vi "_Set 1 DAC Value.vi"(1 "DAC":u32, 3 "Ch#":u8) -> (0 "PIC Monitor":u8)   [LabVIEW 2015]
uses:
  Type/_FPGA Chip Type.ctl
  <vilib>/rvi/eio/common/nirviEmuTemplateMethod_errors.vi
  <vilib>/rvi/Memory/Memory_Emulation/nirvimemoryEmulation.vi
  <vilib>/rvi/Memory/Memory_Emulation/nirvimemoryFastEmulation.vi
  <vilib>/rvi/DataTransferAndStorage/Container/Common/niFpgaContainerGetUniqueNameForEmu.vi
  <vilib>/rvi/Memory/Memory_Emulation/niFpgaMemoryEmulationCacheClearOnFirstRun.vi
  <vilib>/rvi/Memory/Memory_Emulation/nirvimemoryEmulationManagerCache_MakeExclusive.vi
  <vilib>/rvi/Memory/Memory_Emulation/niFpgaMemoryEmulationValidateCache.vi
  <vilib>/rvi/Memory/Memory_Emulation/nirvimemoryEmulationManagerCache_InsertValue.vi
  <vilib>/Utility/error.llb/Clear Errors.vi
  <vilib>/rvi/Memory/Memory_Emulation/nirvimemoryEmulationManagerCache_ReleaseExclusive.vi
  <vilib>/rvi/Memory/Memory_Emulation/nirvimemoryEmulationManagerCache_GetValue.vi
  <vilib>/rvi/Emulation/niFpgaEmulationIsFPGAContextNoSignature.vi
  <vilib>/rvi/Emulation/niFpgaSctlEmulationGetInTimedLoop.vi
  <vilib>/rvi/Memory/Memory_Emulation/nirvimemoryEmulationManagerCache_SetValue.vi
  <vilib>/rvi/Emulation/niFpgaSctlEmulationResourceMgr.vi
  <vilib>/eio/EIONode/EIONode.xnode
  <vilib>/rvi/DataTransferAndStorage/Container/XNode/niFpgaContainer.xnode
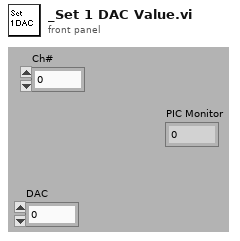
[diagram p1: front panel]
types:
  T1 = typedef "_FPGA Chip Type.ctl" = enum8{"None", "ADC1", "ADC2", "ADC3", "ADC4", "ADC5", "ADC6", "ADC7", "ADC8", "ADC9", "ADC10", "ADC11", "ADC12", "ADC13", "DAC1", "DAC2", "DAC3", "DAC4", "DAC5", "LENS1", "LENS2", "LENS3", "LENS4", "LENS5", "LENS6", "LENS7", "MASS1", "MASS2", "MASS3", "MASS4", "MASS5", "OSC1", "OSC2", "OSC3", "LATCH1", "LATCH2", "LATCH3", "LATCH4", "PIC1", "PIC2", "PIC3", "PIC4"}
  T2 = cluster{"Boolean array[0]":bool, "Boolean array[1]":bool, "Boolean array[2]":bool, "Boolean array[3]":bool, "Boolean array[4]":bool, "Boolean array[5]":bool, "Boolean array[6]":bool, "Boolean array[7]":bool, "Boolean array[8]":bool, "Boolean array[9]":bool, "Boolean array[10]":bool, "Boolean array[11]":bool, "Boolean array[12]":bool, "Boolean array[13]":bool, "Boolean array[14]":bool, "Boolean array[15]":bool, "Boolean array[16]":bool, "Boolean array[17]":bool, "Boolean array[18]":bool, "Boolean array[19]":bool, "Boolean array[20]":bool, "Boolean array[21]":bool, "Boolean array[22]":bool, "Boolean array[23]":bool, "Boolean array[24]":bool, "Boolean array[25]":bool, "Boolean array[26]":bool, "Boolean array[27]":bool, "Boolean array[28]":bool, "Boolean array[29]":bool, "Boolean array[30]":bool, "Boolean array[31]":bool}
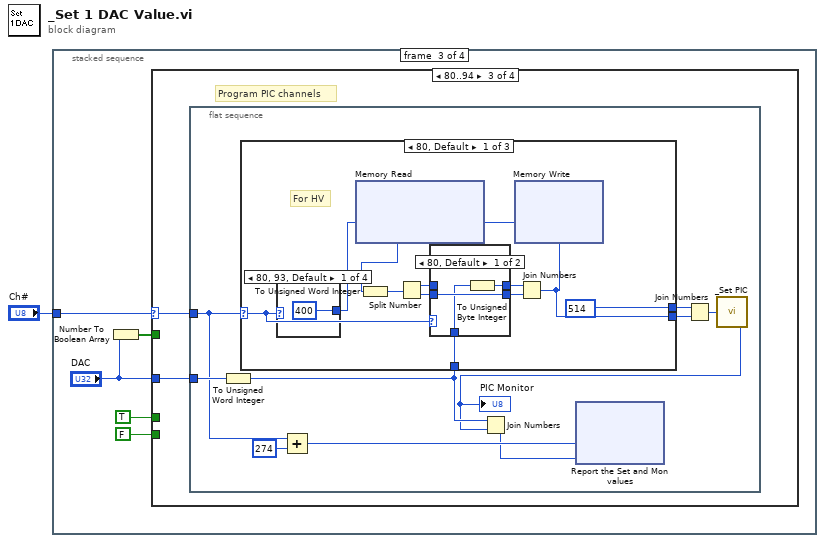
[diagram p0: block diagram]
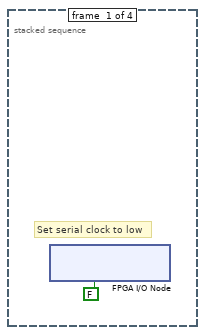
[diagram p2: hidden frame]
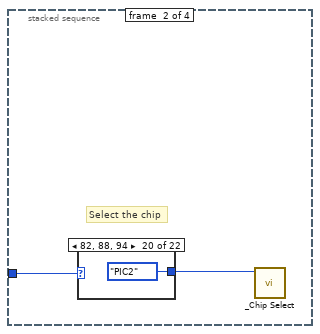
[diagram p3: hidden frame]
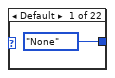
[diagram p4: hidden frame]
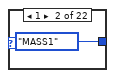
[diagram p5: hidden frame]
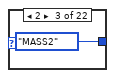
[diagram p6: hidden frame]
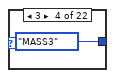
[diagram p7: hidden frame]
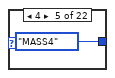
[diagram p8: hidden frame]
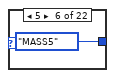
[diagram p9: hidden frame]
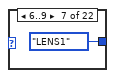
[diagram p10: hidden frame]
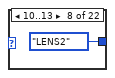
[diagram p11: hidden frame]
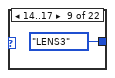
[diagram p12: hidden frame]
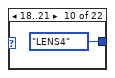
[diagram p13: hidden frame]
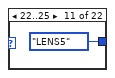
[diagram p14: hidden frame]
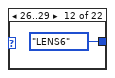
[diagram p15: hidden frame]
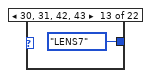
[diagram p16: hidden frame]
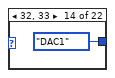
[diagram p17: hidden frame]
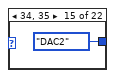
[diagram p18: hidden frame]
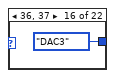
[diagram p19: hidden frame]
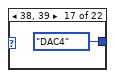
[diagram p20: hidden frame]
diagram:
  n1 = stacked-sequence {
    tunnel: "Ch#" -> [_ w3 w30 _]
    frame #0 {
      # "Set serial clock to low"
      n2 = xnode "FPGA I/O Node"("Digtal IO/DIO9"=FALSE ("Port1/DIO0")) -> ()  [unwired: 1 in, 1 out]
    }
    frame #1 {
      # "Select the chip"
      n3 = case shown="82, 88, 94" w3 {
        tunnel: [_FPGA_Chip_Type."None" ("ChipType") _FPGA_Chip_Type."MASS1" ("ChipType") _FPGA_Chip_Type."MASS2" ("ChipType") _FPGA_Chip_Type."MASS3" ("ChipType") _FPGA_Chip_Type."MASS4" ("ChipType") _FPGA_Chip_Type."MASS5" ("ChipType") _FPGA_Chip_Type."LENS1" ("ChipType") _FPGA_Chip_Type."LENS2" ("ChipType") _FPGA_Chip_Type."LENS3" ("ChipType") _FPGA_Chip_Type."LENS4" ("ChipType") _FPGA_Chip_Type."LENS5" ("ChipType") _FPGA_Chip_Type."LENS6" ("ChipType") _FPGA_Chip_Type."LENS7" ("ChipType") _FPGA_Chip_Type."DAC1" ("ChipType") _FPGA_Chip_Type."DAC2" ("ChipType") _FPGA_Chip_Type."DAC3" ("ChipType") _FPGA_Chip_Type."DAC4" ("ChipType") _FPGA_Chip_Type."DAC5" ("ChipType") _FPGA_Chip_Type."PIC1" ("ChipType") _FPGA_Chip_Type."PIC2" ("ChipType") _FPGA_Chip_Type."PIC3" ("ChipType") _FPGA_Chip_Type."PIC4" ("ChipType")] -> w4
        frame Default {
        }
        frame 1 {
        }
        frame 2 {
        }
        frame 3 {
        }
        frame 4 {
        }
        frame 5 {
        }
        frame 6..9 {
        }
        frame 10..13 {
        }
        frame 14..17 {
        }
        frame 18..21 {
        }
        frame 22..25 {
        }
        frame 26..29 {
        }
        frame 30, 31, 42, 43 {
        }
        frame 32, 33 {
        }
        frame 34, 35 {
        }
        frame 36, 37 {
        }
        frame 38, 39 {
        }
        frame 40, 41 {
        }
        frame 80, 81, 87, 93 {
        }
        frame 82, 88, 94 {
        }
        frame 83, 84, 89, 91 {
        }
        frame 85, 86, 90, 92 {
        }
      }
      n4 = call "_Chip Select.vi"("ChipType"=w4) -> ()  [unwired: 1 in, 6 out]
    }
    frame #2 {
      n5 = Number To Boolean Array(number="DAC") -> (Boolean array=w29:bool[])
      n6 = case shown="80..94" w30 {
        selector: w30 -> [w32 w69 w96 _]
        tunnel: w29 -> [w35 w74 _ _]
        tunnel: TRUE -> [w34 w72 _ _]
        tunnel: FALSE -> [w33 w71 _ _]
        tunnel: "DAC" -> [_ _ w95 _]
        frame 1..31, 42, 43 {
          n7 = flat-sequence {
            tunnel: w35 -> [w36]
            tunnel: w32 -> [w61]
            tunnel: w34 -> [w38]
            tunnel: w33 -> [w37]
            frame #0 {
              # "D17"
              # "D0"
              # "WR"
              # "A1"
              # "A0"
              # "2 Address bits"
              # "Program Parallel DAC Data"
              n8 = case shown="1, Default" w61 {
                tunnel: w38 -> [w62 _ w65 w66]
                tunnel: w37 -> [_ w63 w64 w67]
                tunnel: [w62 w63 w65 w67] -> w40
                tunnel: [w62 w63 w64 w66] -> w39
                frame 1, Default {
                  # "A = 3"
                }
                frame 6, 10, 14, 18, 22, 26, 30 {
                  # "A = 0"
                }
                frame 7, 11, 15, 19, 23, 27, 31 {
                  # "A = 1"
                }
                frame 8, 12, 16, 20, 24, 28, 42 {
                  # "A = 2"
                }
              }
              n9 = call "Wait"("Count(Ticks)"=u8 3) -> ()  [unwired: 1 out]
              n10 = Array To Cluster(array=w36) -> (cluster=w42:T2)
              n11 = Unbundle By Name(w42) -> ("Boolean array[0]"=w43:bool, "Boolean array[1]"=w44:bool, "Boolean array[2]"=w45:bool, "Boolean array[3]"=w46:bool, "Boolean array[4]"=w47:bool, "Boolean array[5]"=w48:bool, "Boolean array[6]"=w49:bool, "Boolean array[7]"=w50:bool, "Boolean array[8]"=w51:bool, "Boolean array[9]"=w52:bool, "Boolean array[10]"=w53:bool, "Boolean array[11]"=w54:bool, "Boolean array[12]"=w55:bool, "Boolean array[13]"=w56:bool, "Boolean array[14]"=w57:bool, "Boolean array[15]"=w58:bool, "Boolean array[16]"=w59:bool, "Boolean array[17]"=w60:bool)
              n12 = xnode "FPGA I/O Node"("Digtal IO/DIO42"=w43, "Digtal IO/DIO41"=w44, "Digtal IO/DIO40"=w45, "Digtal IO/DIO39"=w46, "Digtal IO/DIO38"=w47, "Digtal IO/DIO37"=w48, "Digtal IO/DIO36"=w49, "Digtal IO/DIO35"=w50, "Digtal IO/DIO34"=w51, "Digtal IO/DIO32"=w52, "Digtal IO/DIO31"=w53, "Digtal IO/DIO30"=w54, "Digtal IO/DIO29"=w55, "Digtal IO/DIO28"=w56, "Digtal IO/DIO27"=w57, "Digtal IO/DIO26"=w58, "Digtal IO/DIO25"=w59, "Digtal IO/DIO24"=w60, "Digtal IO/DIO62"=w40, "Digtal IO/DIO61"=w39, "Digtal IO/DIO64"=w37) -> ()  [unwired: 21 in, 21 out]
            }
            frame #1 {
              # "Reset WR bit"
              n13 = xnode "FPGA I/O Node"("Digtal IO/DIO64"=TRUE) -> ()  [unwired: 1 in, 1 out]
            }
          }
        }
        frame 32..41 {
          # "Serial DAC updated immediately without waiting for LDAC"
          # "Transmit the last bit first"
          # "4 Control bits"
          # "Remove the last 16 bits"
          # "R0"
          # "PWR"
          # "SPD"
          # "R1"
          # "Program Serial DAC Data"
          n14 = flat-sequence {
            tunnel: w72 -> [w81]
            tunnel: w71 -> [w80]
            tunnel: w70 -> [w79]
            frame #0 {
              n15 = call "_Update Serial DAC.vi"() -> ()  [unwired: 4 in, 4 out]
            }
            frame #1 {
              n16 = for {
                shift-right: [w83] -> w82
                shift-left: w80 -> [w84]
                tunnel: w79 -> [w83] mode=indexing
                tunnel: w81 -> [w85]
                n17 = flat-sequence {
                  tunnel: w85 -> [w87]
                  tunnel: w84 -> [w86]
                  tunnel: w83 -> [w88]
                  frame #0 {
                    n18 = call "_Update Serial DAC.vi"("DIN (F)"=w86, "Clock (F)"=w87) -> ()  [unwired: 2 in, 4 out]
                  }
                  frame #1 {
                    n19 = call "_Update Serial DAC.vi"("DIN (F)"=w88) -> ()  [unwired: 3 in, 4 out]
                  }
                }
              }
              n20 = call "_Update Serial DAC.vi"("DIN (F)"=w82, "Clock (F)"=w81) -> ()  [unwired: 2 in, 4 out]
            }
          }
          n21 = case shown="32, 34, 36, 38, 40" w69 {
            tunnel: [w91 w94] -> w75
            tunnel: w72 -> [w90 w93]
            tunnel: w71 -> [w89 w92]
            frame 33, Default {
              # "Update DAC B"
              n22 = Build Array(w89, w89, w90, w89) -> (w91:bool[])
            }
            frame 32, 34, 36, 38, 40 {
              # "Update DAC A"
              n23 = Build Array(w92, w92, w93, w93) -> (w94:bool[])
            }
          }
          n24 = Array Subset(array=w74, length=16 ("index")) -> (w76:bool[])  [unwired: 1 in]
          n25 = Replace Array Subset(array=w76, new element=w75, index=12) -> (w73:bool[])
          n26 = Reverse 1D Array(array=w73) -> (reversed array=w70:bool[])
        }
        frame 80..94 {
          # "Program PIC channels"
          n27 = flat-sequence {
            tunnel: w96 -> [w97]
            tunnel: w95 -> [w101]
            frame #0 {
              n28 = To Unsigned Word Integer(number=w101) -> (unsigned 16bit integer=w100:u16)
              n29 = case shown="80, Default" w97 {
                selector: w97 -> [w117 _ _]
                tunnel: [i16 514 i16 257 i16 771] -> w106
                tunnel: [w114 w128 u16 0] -> w104
                tunnel: w100 -> [w115 w128 _]
                frame 80, Default {
                  # "For HV"
                  n30 = case shown="80, 93, Default" w117 {
                    tunnel: [u16 400 u16 401 u16 402 u16 403] -> w111
                    frame 80, 93, Default {
                    }
                    frame 82, 94 {
                    }
                    frame 83, 91 {
                    }
                    frame 85, 92 {
                    }
                  }
                  n31 = xnode ("Memory Read")("Address"=w111) -> ("Data"=w108:u32)  [unwired: 1 in, 1 out]
                  n32 = To Unsigned Word Integer(number=w108) -> (unsigned 16bit integer=w107:u16)
                  n33 = Split Number(x=w107) -> (hi(x)=w113:u8, lo(x)=w112:u8)
                  n34 = case shown="80, Default" w117 {
                    tunnel: w113 -> [_ w123]
                    tunnel: w112 -> [w120 _]
                    tunnel: [w120 w121] -> w109
                    tunnel: [w118 w123] -> w110
                    tunnel: w115 -> [w119 w122]
                    frame 80, Default {
                      n35 = To Unsigned Byte Integer(number=w119) -> (unsigned 8bit integer=w118:u8)
                    }
                    frame 91..94 {
                      n36 = To Unsigned Byte Integer(number=w122) -> (unsigned 8bit integer=w121:u8)
                    }
                  }
                  n37 = Join Numbers(hi=w110, lo=w109) -> ((hi.lo)=w114:u16)
                  n38 = xnode ("Memory Write")("Address"=w111, "Data"=w114) -> ()  [unwired: 1 in, 1 out]
                }
                frame 81, 84, 86 {
                  # "for Temp"
                }
                frame 87..90 {
                  # "for Probe ID"
                }
              }
              n39 = Add(x=w97, y=u16 274) -> (x+y=w102:u16)
              n40 = Join Numbers(hi=w106, lo=w104) -> ((hi.lo)=w105:u32)
              n41 = call "_Set PIC.vi"("Data"=w105) -> ("PIC Monitor"=w99:u16)
              "PIC Monitor" <- w99
              n42 = Join Numbers(hi=w100, lo=w99) -> ((hi.lo)=w98:u32)
              n43 = xnode "Report the Set and Mon values"("Address"=w102, "Data"=w98) -> ()  [unwired: 1 in, 1 out]
            }
          }
        }
        frame Default {
          # "Unknow channel ID, do nothing"
        }
      }
    }
    frame #3 {
      # "Cancel the chip select"
      n44 = xnode "FPGA I/O Node"("Digtal IO/DIO9"=FALSE ("Port1/DIO0")) -> ()  [unwired: 1 in, 1 out]
      n45 = call "_Chip Select.vi"() -> ()  [unwired: 2 in, 6 out]
    }
  }
